vi "Read DCV_DCI.vi"(6 "wait for reply (T)":bool=TRUE, 8 "error in":errorcluster, 11 "Sets to Display":u16(ring) items=["1st Display", "2nd Display", "1st & 2nd Display"]) -> (0 "error out":errorcluster, 1 "timed out?":bool, 2 "DCI":dbl, 3 "DCV":dbl)   [LabVIEW 2018, in "DMM Module.lvlib"]
doc: "Read DCV, DCI dual measurements\n_____\nCreated using DQMH Event Scripter 6.0.0.122."
uses:
  DMM Module.lvlib
  Read DCV_DCI Argument--cluster.ctl
  Read DCV_DCI (Reply Payload)--cluster.ctl
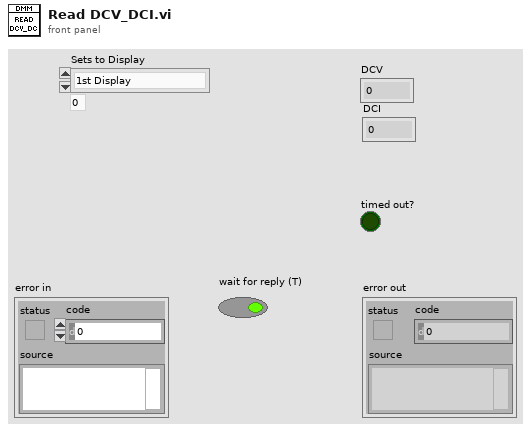
[diagram p1: front panel]
types:
  T1 = typedef "DMM Module.lvlib/Read DCV_DCI Argument--cluster.ctl" = cluster{"Wait Notifier":refnum<notifier>, "wait for reply":bool, "Sets to Display":u16}
  T2 = typedef "DMM Module.lvlib/Request Events--cluster.ctl" = cluster{"Stop Module":refnum<user-event>, "Do Something Else":refnum<user-event>, "Do Something Else and Wait for Reply":refnum<user-event>, "Show Panel":refnum<user-event>, "Hide Panel":refnum<user-event>, "Get Module Execution Status":refnum<user-event>, "Show Diagram":refnum<user-event>, "DMM init":refnum<user-event>, "config channel":refnum<user-event>, "Read DCV_DCI":refnum<user-event>}
  T3 = typedef "DMM Module.lvlib/Read DCV_DCI (Reply Payload)--cluster.ctl" = cluster{"DCV":dbl, "DCI":dbl, "Read DCV_DCI_error":errorcluster}
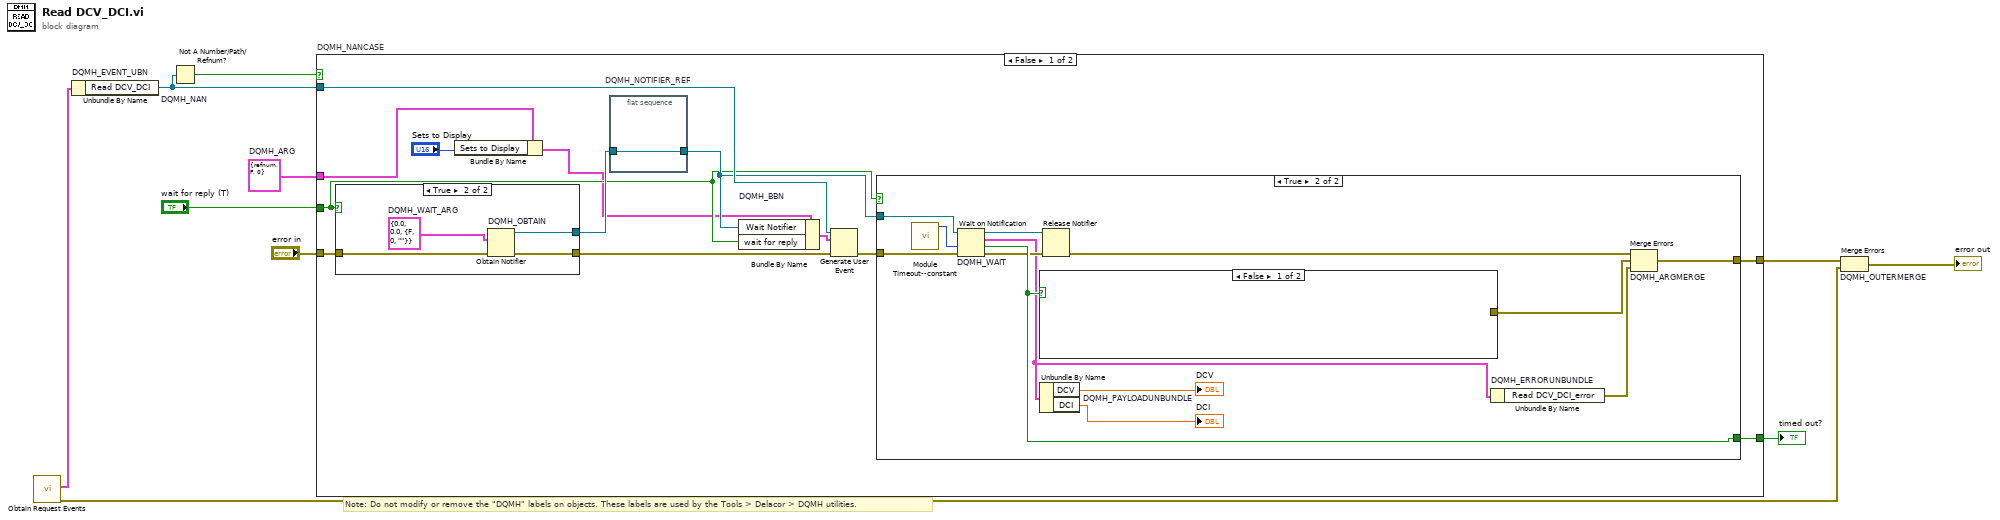
[diagram p0: block diagram]
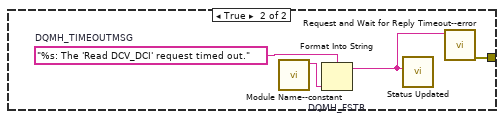
[diagram p3: hidden frame]
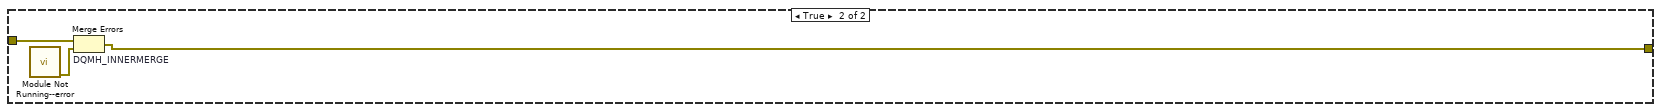
[diagram p5: hidden frame]
diagram:
  w4 = T1 {"Wait Notifier"=refnum, "wait for reply"=FALSE, "Sets to Display"=0}  # DQMH_ARG
  # "Note: Do not modify or remove the \"DQMH\" labels on objects. These labels are used by the Tools > Delacor > DQMH utilities."
  n1 = call "Obtain Request Events.vi"() -> ("error out"=w2:errorcluster, "DMM Module Request Events"=w1:T2)  [unwired: 10 in]
  n2 = Unbundle By Name "DQMH_EVENT_UBN"(w1) -> ("Read DCV_DCI"=w8:refnum<user-event>)
  n3 = Not A Number/Path/Refnum? "DQMH_NAN"(number/path/refnum=w8) -> (NaN/Path/Refnum?=w7:bool)
  n4 = case "DQMH_NANCASE" shown="False" w7 {
    tunnel: "error in" -> [w23 w50]
    tunnel: w8 -> [w21 _]
    tunnel: [w18 w49] -> w5
    tunnel: [w19 _] -> w6
    tunnel: w4 -> [w11 _]
    tunnel: "wait for reply (T)" -> [w14 _]
    frame False {
      n5 = case shown="True" w14 {
        tunnel: w23 -> [w43 w47]
        tunnel: [w43 w46] -> w20
        tunnel: [_ w44] -> w16
        frame False {
        }
        frame True {
          w45 = T3 {"DCV"=0.0, "DCI"=0.0, "Read DCV_DCI_error"={"status"=FALSE, "code"=0, "source"=""}}  # DQMH_WAIT_ARG
          n6 = Obtain Notifier "DQMH_OBTAIN"(notification data type=w45, error in (no error)=w47) -> (notifier out=w44:refnum<notifier>, error out=w46:errorcluster)  [unwired: 2 in, 1 out]
        }
      }
      n7 = Bundle By Name(cluster=w11, "Sets to Display"="Sets to Display") -> (w12:T1)
      n8 = flat-sequence "DQMH_NOTIFIER_REF" {
        tunnel: w16 -> [w24]
        tunnel: [w24] -> w15
        frame #0 {
        }
      }
      n9 = Bundle By Name "DQMH_BBN"(cluster=w12, "Wait Notifier"=w15, "wait for reply"=w14) -> (w17:T1)
      n10 = Generate User Event(user event=w21, event data cluster=w17, error in=w20) -> (error out=w22:errorcluster)  [unwired: 1 in, 1 out]
      n11 = case shown="True" w14 {
        tunnel: w22 -> [w25 w38]
        tunnel: w15 -> [_ w37]
        tunnel: [_ w35] -> w19
        tunnel: [w25 w34] -> w18
        frame False {
        }
        frame True {
          n12 = call "Module Timeout--constant.vi"() -> ("Module Timeout"=w28:i32)  [unwired: 11 in]
          n13 = Wait on Notification "DQMH_WAIT"(notifier=w37, timeout in ms (-1)=w28, error in (no error)=w38) -> (notifier out=w36:refnum<notifier>, notification=w29:T3, timed out?=w35:bool, error out=w33:errorcluster)  [unwired: 1 in]
          n14 = case shown="False" w35 {
            tunnel: [_ w40] -> w30
            frame False {
            }
            frame True {
              w42 = "%s: The 'Read DCV_DCI' request timed out."  # DQMH_TIMEOUTMSG
              n15 = call "Module Name--constant.vi"() -> ("Module Name"=w39:string)  [unwired: 11 in]
              n16 = Format Into String "DQMH_FSTR"(format string=w42, w39) -> (resulting string=w41:string)  [unwired: 2 in, 1 out]
              n17 = call "Status Updated.vi"("Status"=w41) -> ()  [unwired: 10 in, 1 out]
              n18 = call "Request and Wait for Reply Timeout--error.vi"("Error Message"=w41) -> ("error out"=w40:errorcluster)  [unwired: 10 in]
            }
          }
          n19 = Unbundle By Name "DQMH_PAYLOADUNBUNDLE"(w29) -> ("DCV"=→"DCV":dbl, "DCI"=→"DCI":dbl)
          n20 = Release Notifier(notifier=w36, error in (no error)=w33) -> (error out=w32:errorcluster)  [unwired: 1 in, 2 out]
          n21 = Unbundle By Name "DQMH_ERRORUNBUNDLE"(w29) -> ("Read DCV_DCI_error"=w31:errorcluster)
          n22 = Merge Errors "DQMH_ARGMERGE"(w32, w30, w31) -> (w34:errorcluster)
        }
      }
    }
    frame True {
      n23 = call "Module Not Running--error.vi"() -> ("error out"=w48:errorcluster)  [unwired: 11 in]
      n24 = Merge Errors "DQMH_INNERMERGE"(w50, w48) -> (w49:errorcluster)
    }
  }
  "timed out?" <- w6
  n25 = Merge Errors "DQMH_OUTERMERGE"(w5, w2) -> (→"error out":errorcluster)
